vi "AOD Control (FPGA).vi"() -> ()   [LabVIEW 2014]
uses:
  FPGAState.ctl
  AODCalibration.ctl
  CoordinateSettings.ctl
  <vilib>/Platform/TimedLoop/XDataNode/timing_clust.ctl
  <vilib>/Platform/TimedLoop/XDataNode/nitl_modes.ctl
  <vilib>/Platform/TimedLoop/XDataNode/wakeup.ctl
  <vilib>/rvi/Emulation/niFpgaSctlEmulationGetInTimedLoop.vi
  <vilib>/rvi/Emulation/niFpgaEmulationReportErrorSimple.vi
  <vilib>/rvi/Emulation/niFpgaGetClockAttributes.vi
  <vilib>/rvi/Emulation/niFpgaCriticalErrorInLSC.vi
  <vilib>/rvi/eio/common/nirviEmuTemplateMethod_errors.vi
  <vilib>/rvi/Emulation/niFpgaProcessEmulError.vi
  <vilib>/rvi/interface/RandomDataEmulation/niFpgaRandomDataHandleErrors.vi
  <vilib>/Platform/TimedLoop/XDataNode/XDataNode.xnode
  <vilib>/eio/EIONode/EIONode.xnode
  <vilib>/rvi/DataTransferAndStorage/Container/XNode/niFpgaContainer.xnode
  <vilib>/rvi/interface/RandomDataEmulation/nirviRandomDataFpgaReadWriteTemplate.vi
  <vilib>/Platform/TimedLoop/XDataNode/XDNodeRunTimeDep.lvlib
  <vilib>/rvi/occurrence/nirviOccurrence.lvlib
  <vilib>/rvi/Analysis/measure/butterworth/XNode/niFpgaButterworthFilter.xnode
panel:
  out "Status.MotionCorrectionChFull":bool
  out "Status.RelativeRate":u64
  out "Status.Update IO Missing":bool
  out "Status.Last Point":bool
  out "Status.All Samples":bool
  out "Status.AcqState":enum16{"Idling", "Acquiring"}(ring)
  out "Status.TemporalChFull":bool
  out "Status.MotionChFull":bool
  out "Status.ImChFull":bool
  out "Status.BufferedPoints":i32
  out "Status.Sequencer":T1
  out "Status.Initialized":bool
  out "Status.RepNum":u32
  out "Status.Mode":enum16{"Points", "Volume", "Idle"}(ring)
  out "Status.ScanDone":bool
  out "Status.Armed":bool
  out "Status.ScanUpdateIO":bool
  out "Status.Writing":bool
  out "Status.PointTime":u32
  out "Status.PointNum":u32
  out "Status.Sequencing error":bool
  in  "OutOffset.Z":i32
  in  "OutOffset.Y":i32
  in  "OutOffset.X":i32
  in  "InOffset.Z":i32
  in  "InOffset.Y":i32
  in  "InOffset.X":i32
  in  "Setup.DataSource":i16
  in  "Setup.BitShift":i16
  in  "Setup.Downsample":u32=1000
  in  "Setup.Timeout":i32=40000000
  out "Filtered Data":i32[](array[numeric])
  in  "scaled coefficients":i32[](array[numeric])=[-807278098, 1858776710, 5560803, -954717605, 2004472733, 5996674]
  out "Debug.FilterTime":u32
  out "Debug.WriteTime":u32
  out "Debug.Sequencing offset":u32
  in  "Debug.Data":i16
  out "Debug.Settings":T2 {"YLP_RR" format="%x"; "YLP_FR" format="%x"; "YHP_RR" format="%x"; "YHP_FR" format="%x"; "XLP_RR" format="%x"; "XLP_FR" format="%x"; "XHPstart" format="%x"; "XHPend" format="%x"; "XLPstart" format="%x"; "XLPend" format="%x"; "YHPstart" format="%x"; "YHPend" format="%x"; "YLPstart" format="%x"; "YLPend" format="%x"; "XHP_RR" format="%x"; "XHP_FR" format="%x"}
  out "Debug.PMT_Unpacked_backlog":u32
  out "Debug.PMT_Data_backlog":u32
  in  "Debug.FinishedSettingSize":i16=3
  in  "Debug.FinishedSetting":cluster{"Address":u8, "Value":u32}[](array[cluster])=[{"Address"=0, "Value"=246}, {"Address"=4, "Value"=0}, {"Address"=5, "Value"=0}, {"Address"=0, "Value"=0}, {"Address"=0, "Value"=0}] {"Address" format="%x"; "Value" format="%x"}
  in  "Debug.Coordinate":T3
  in  "Debug.SetCoordinate":bool
  out "Debug.AcqDivCount":u32
  out "Debug.PMT_Samples":u32
  out "Debug.MainLoopCount":i32
  in  "Debug.UpdateIO":bool
  out "Debug.PMT Array":i32[](array[numeric])
  in  "Debug.P":bool
  in  "Debug.Point":cluster{"X":i32, "Y":i32, "Z":i32}
  in  "Debug.Write Point":bool
  out "Error.Sequencer":bool
  out "Error.UpdateIOTimeout":bool
  out "Error.Serial error":bool
  out "Error.OutOfRange":bool
  out "Error.Bad Coordinate":bool
  out "Status.WaitingDownsamplerEnd":bool
  in  "Comm.P delay":u32=10
  in  "Comm.P high":u32=10
  in  "Comm.Pause":u32
  in  "Comm.WriteSize":i32
  in  "Comm.Write":cluster{"Address":u8, "Value":u32}[](array[cluster])=[{"Address"=0, "Value"=0}, {"Address"=0, "Value"=0}, {"Address"=0, "Value"=0}, {"Address"=0, "Value"=0}, {"Address"=0, "Value"=0}, {"Address"=0, "Value"=0}, {"Address"=0, "Value"=0}, {"Address"=0, "Value"=0}, {"Address"=0, "Value"=0}, {"Address"=0, "Value"=0}, {"Address"=0, "Value"=0}, {"Address"=0, "Value"=0}, {"Address"=0, "Value"=0}, {"Address"=0, "Value"=0}, {"Address"=0, "Value"=0}, {"Address"=0, "Value"=0}, {"Address"=0, "Value"=0}, {"Address"=0, "Value"=0}, {"Address"=0, "Value"=0}, {"Address"=0, "Value"=0}]
  out "Comm.WritenCount":i32
  in  "Comm.Write Register":bool
  in  "Comm.SclkDivider":u32=10
  in  "Comm.CommLines":enum16{"1", "2", "4"}(ring)
  in  "Comm.UpdateIO time":u32=2
  out "Scan.SampleToLoad":u32
  out "Scan.UpdateIO counter":u32
  out "Scan.Downsample Counter":u32
  in  "Scan.NumMotionPoints":u32
  in  "Scan.Motion Increment":u32
  in  "Scan.TotalSamples":u32
  in  "Scan.VolumeSettings":T4={"XStart"=0, "XEnd"=0, "XNum"=1, "YStart"=0, "YEnd"=0, "YNum"=1, "ZStart"=0, "ZEnd"=0, "ZNum"=1} {"ZNum" min=1 max=10000; "YNum" min=1 max=10000; "XNum" min=1 max=10000}
  in  "Scan.NumReps":i32=1
  in  "Scan.NumPoints":u32
  out "Scan.Acquire Samples":u32
  out "Clock100 PLL Unlocked":bool
  out "IO Module\\Initialization Done":bool
  in  "IO Module\\Force Initialization":bool
  in  "IO Module\\Sample Clock Select":u8
  out "IO Module\\Pll Unlocked":bool
  out "Analog Data":i16[](array[numeric])
  in  "AOD.Calibration":T5={"XHP ChirpGain"=1.0, "YHP ChirpGain"=1.0, "XLP ChirpGain"=1.0, "YLP ChirpGain"=1.0}
  in  "AOD.ThrowawaySamples":u16=40
  in  "AOD.LP Center Frequency":u32=858993459 format="%x"
  in  "AOD.HP Center Frequency":u32=805306367 format="%x"
  in  "AOD.Range":u32=214748364 format="%x"
  in  "AOD.BlankSamples":u16=500
  in  "AOD.UpdatesPerPoint":u32=2000
  in  "Control.Points":bool
  in  "Control.Reset":bool
  in  "Control.Abort":bool
  in  "Control.Volume":bool
  in  "Control.Stop":bool
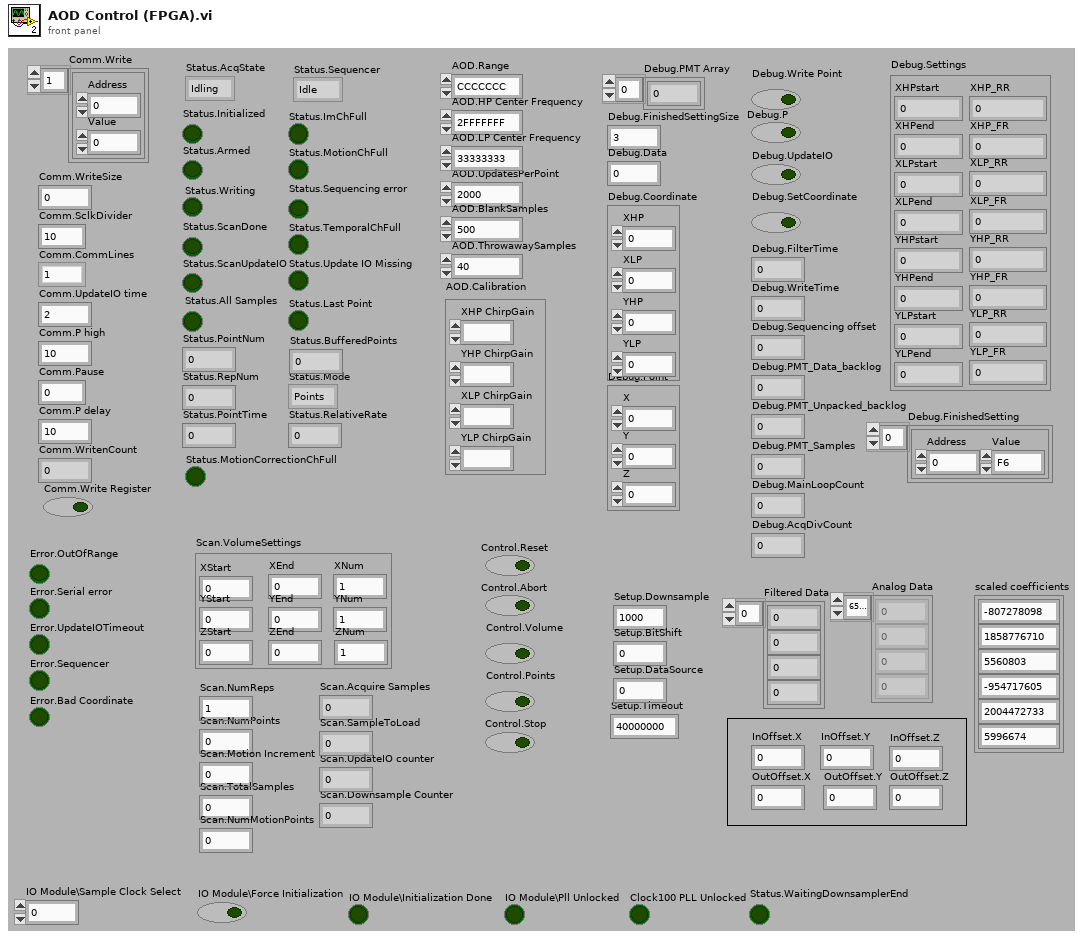
[diagram p1: front panel]
types:
  T1 = typedef "FPGAState.ctl" = enum16{"Idle", "Arm Scan", "Scan", "End Scan"}
  T2 = typedef "CoordinateSettings.ctl" = cluster{"XHPstart":u32, "XHPend":u32, "XLPstart":u32, "XLPend":u32, "YHPstart":u32, "YHPend":u32, "YLPstart":u32, "YLPend":u32, "XHP_RR":u32, "XHP_FR":u32, "XLP_FR":u32, "XLP_RR":u32, "YHP_FR":u32, "YHP_RR":u32, "YLP_FR":u32, "YLP_RR":u32}
  T3 = cluster{"XHP":i32, "XLP":i32, "YHP":i32, "YLP":i32}
  T4 = cluster{"XStart":i32, "XEnd":i32, "XNum":i32, "YStart":i32, "YEnd":i32, "YNum":i32, "ZStart":i32, "ZEnd":i32, "ZNum":i32}
  T5 = typedef "AODCalibration.ctl" = cluster{"XHP ChirpGain":fxp<+/-,16,2>, "YHP ChirpGain":fxp<+/-,16,2>, "XLP ChirpGain":fxp<+/-,16,2>, "YLP ChirpGain":fxp<+/-,16,2>}
  T6 = typedef "XDNodeRunTimeDep.lvlib/timing_clust.ctl" = cluster{"Expected End [f-1]":u64, "Actual End [f-1]":u64, "Finished Late? [f-1]":bool, "Expected End [i-1]":u64, "Actual End [i-1]":u64, "Finished Late? [i-1]":bool, "Expected Start [i]":u64, "Actual Start [i]":u64, "Expected Start [f]":u64, "Actual Start [f]":u64, "Source Name":string, "Structure Name":string, "Period":i64, "Deadline":i64, "Offset":i64, "Start":i64, "Priority":i32, "Timeout":i32, "Mode":T7, "Wakeup Reason":T8, "Error":errorcluster, "Source Type":string, "Secondary Source Type":string, "Global End Time":u64, "Global Start Time":u64, "Frame Duration":u64, "Iteration Duration":u64, "Assigned CPU":i32, "I/O Scan Engine Mode":u32}
  T7 = typedef "XDNodeRunTimeDep.lvlib/nitl_modes.ctl" = enum32{"No Change", "Process missed periods, maintain original phase", "Discard missed periods, maintain original phase", "Process missed periods, ignore original phase", "Discard missed periods, ignore original phase"}
  T8 = typedef "XDNodeRunTimeDep.lvlib/wakeup.ctl" = enum32{"Normal", "Aborted", "Asynchronous wakeup", "Timing source error", "Timed loop error", "Timeout"}
  T9 = cluster{"Scan mode":enum16{"Points", "Volume", "Idle"}, "NumPoints":u32, "NumReps":u32, "Motion Increment":u32, "NumMotionPoints":u32, "VolumeSettings":cluster{"XStart":i32, "XEnd":i32, "XNum":i32, "YStart":i32, "YEnd":i32, "YNum":i32, "ZStart":i32, "ZEnd":i32, "ZNum":i32}}
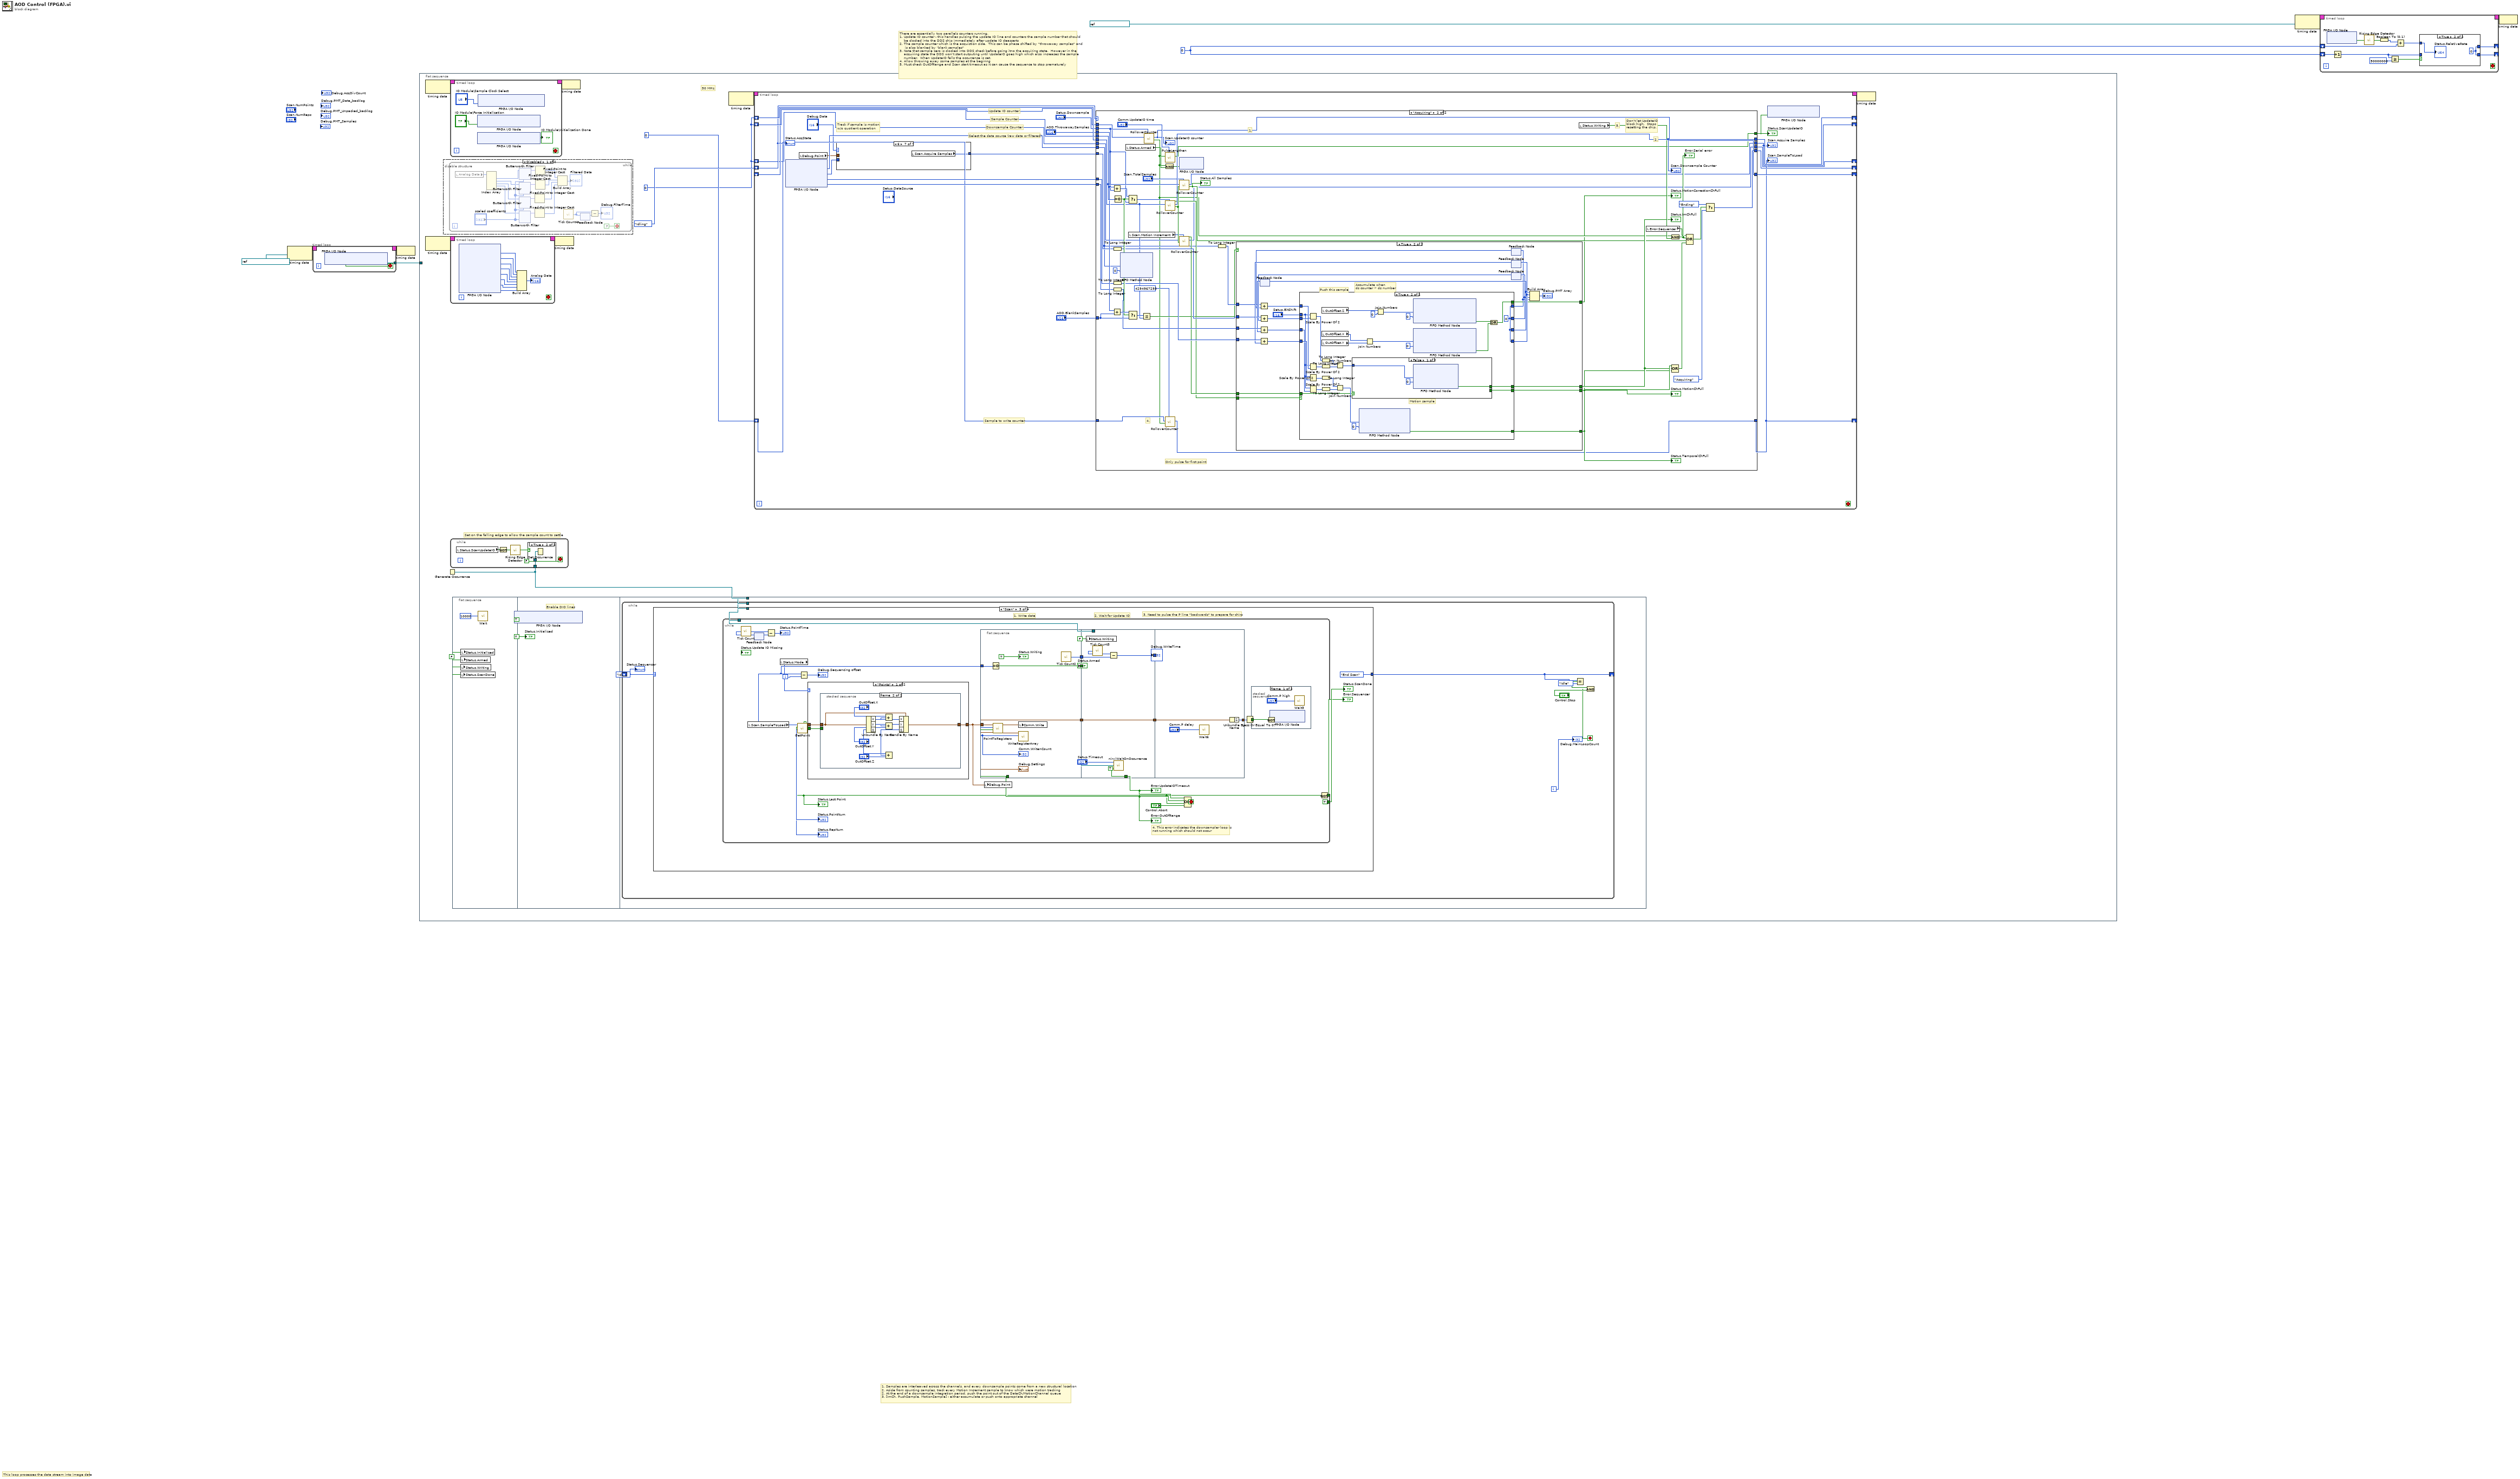
[diagram p0: block diagram]
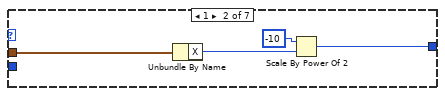
[diagram p6: hidden frame]
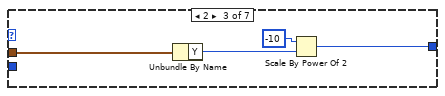
[diagram p7: hidden frame]
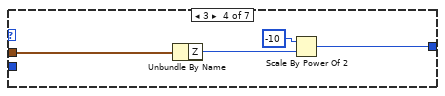
[diagram p8: hidden frame]
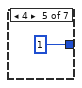
[diagram p9: hidden frame]
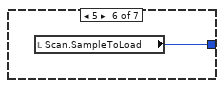
[diagram p10: hidden frame]
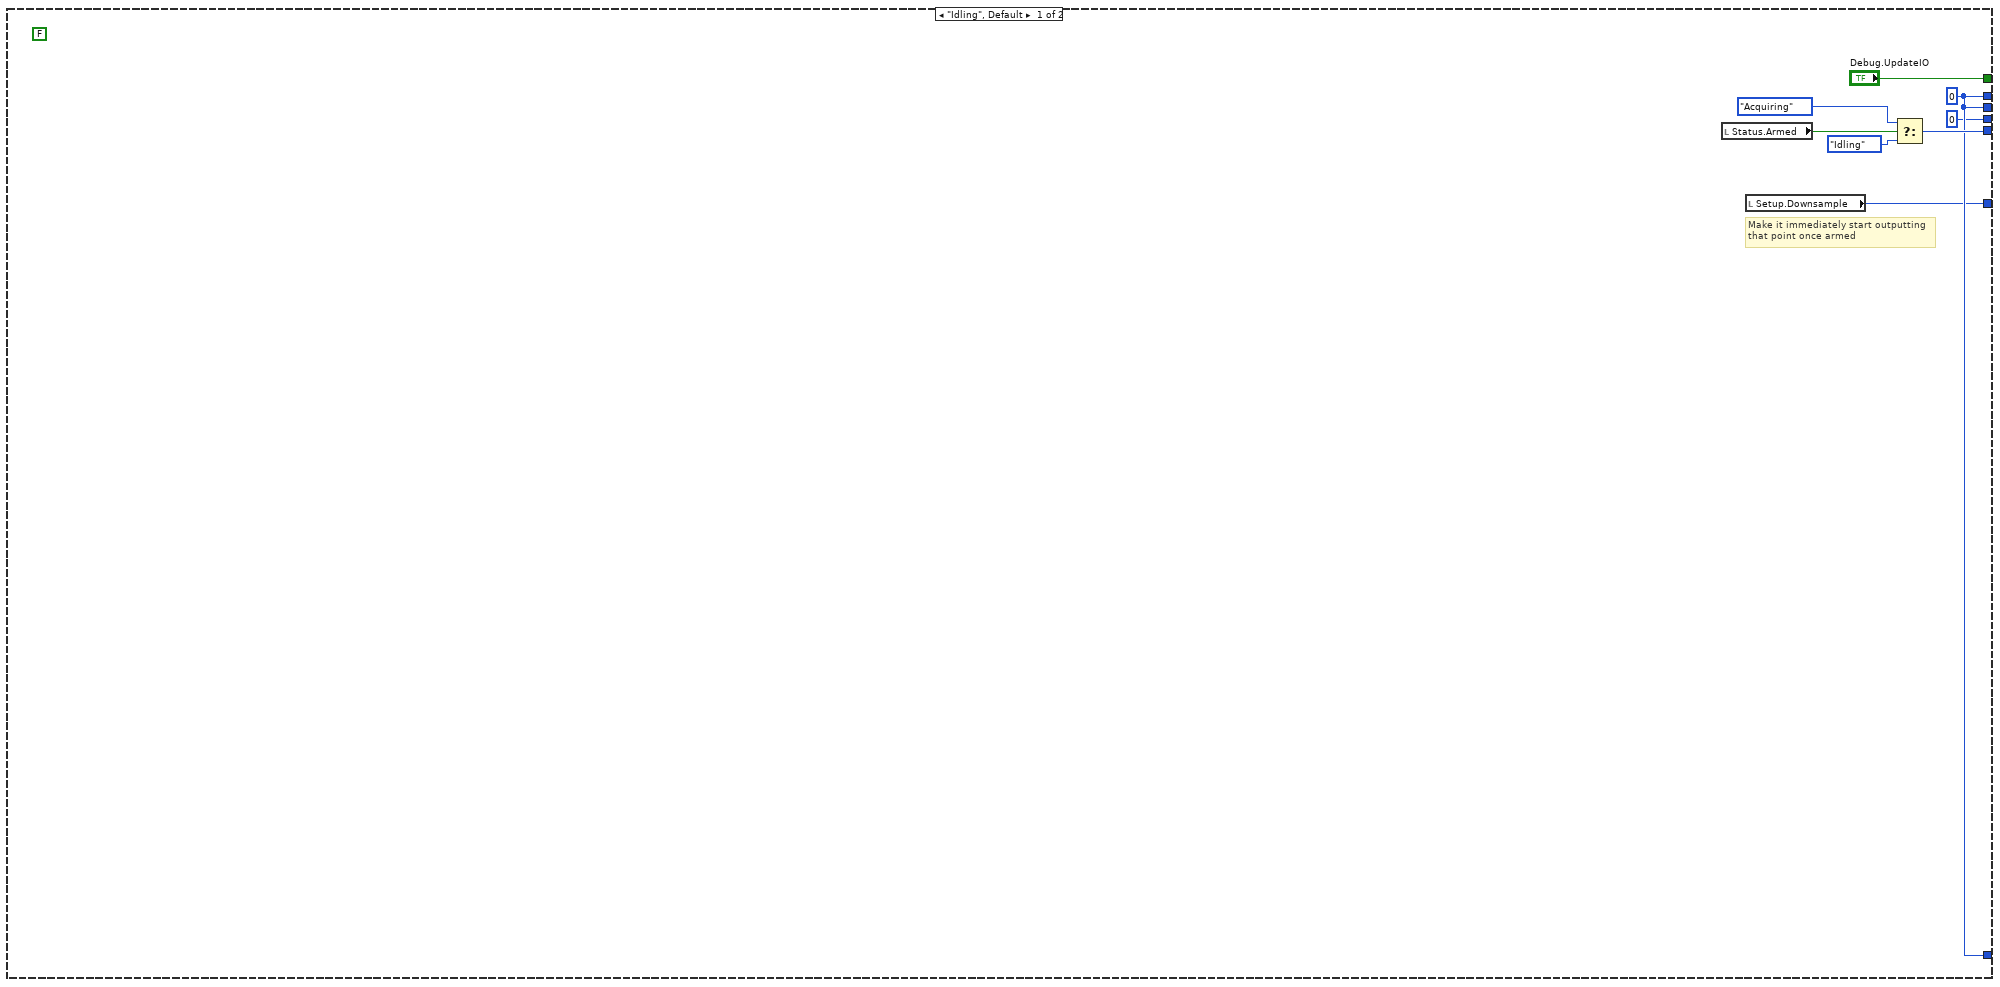
[diagram p11: hidden frame]
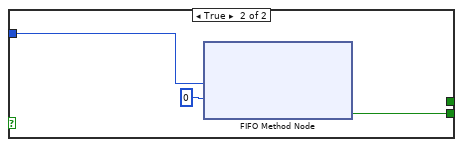
[diagram p14: hidden frame]
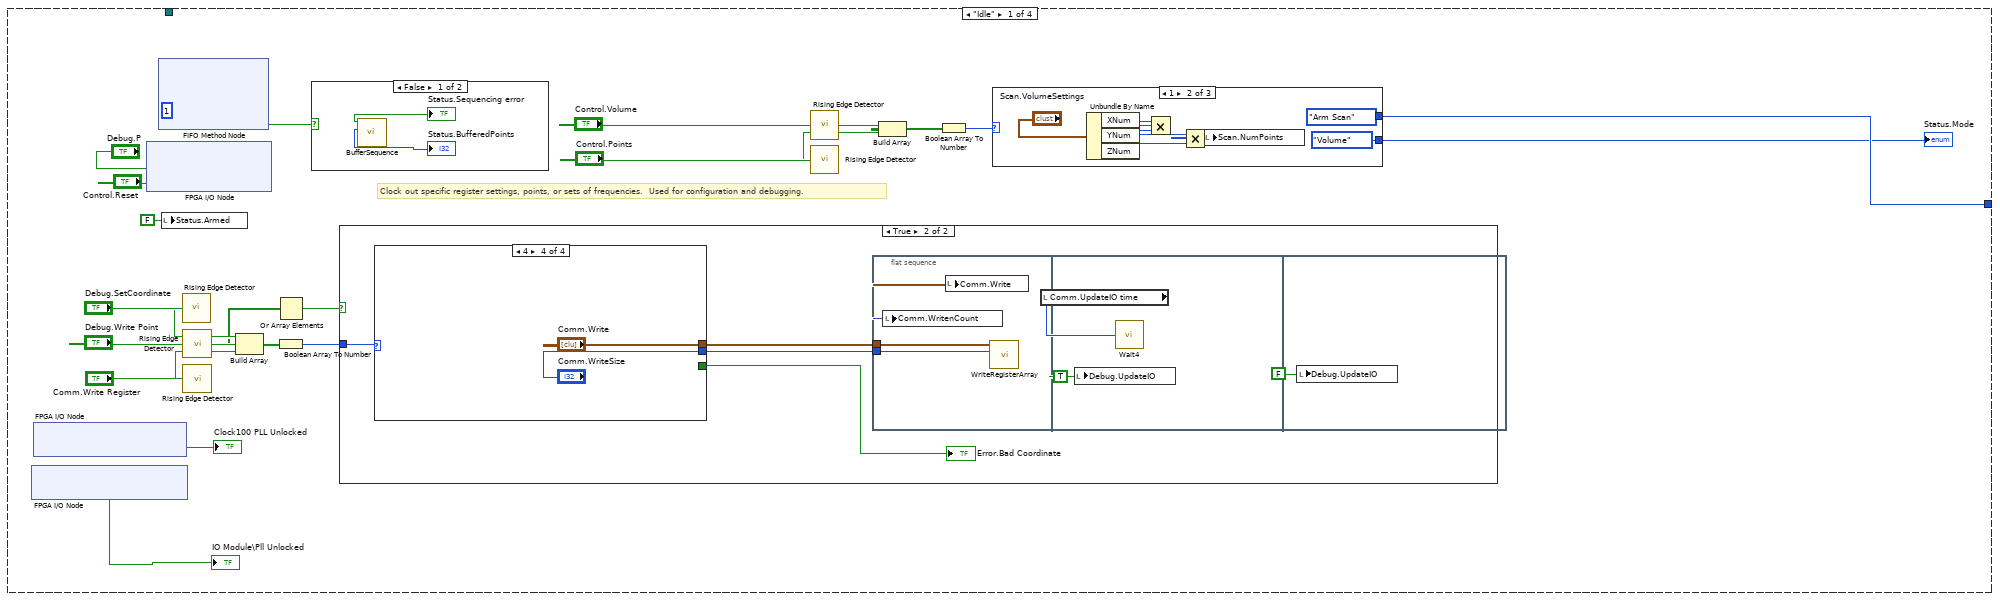
[diagram p15: hidden frame]
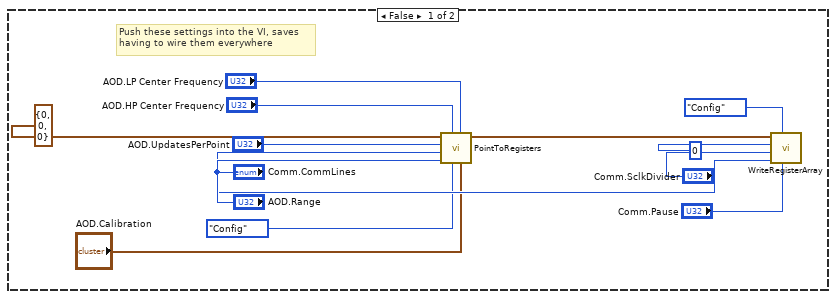
[diagram p17: hidden frame]
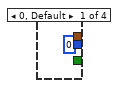
[diagram p18: hidden frame]
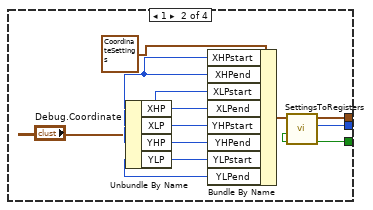
[diagram p19: hidden frame]
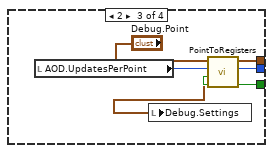
[diagram p20: hidden frame]
diagram:
  w1 = u64 0
  # "There are essentially two parallels counters running.\n1. Update IO counter - this handles pulsing the update IO line and counters the sample number that should\n    be clocked into the DDS chip immediately after update IO deasserts\n2. The sample counter which is the acquistion side.  This can be phase shifted by \"throwaway samples\" and\n     is also blanked by 'blank samples\"\n3. Note that sample zero is clocked into DDS check before going itno the acquiring state.  However in the \n    acquiring state the DDS won't start outputing until UpdateIO goes high which also increases the sample\n    number.  When UpdateIO falls the occurrence is set.\n4. Allow throwing away some samples at the beginng\n5. Must check OutOfRange and Scan start timeout as it can cause the sequence to stop prematurely"
  # "1. Samples are interleaved across the channels, and every downsample points come from a new structural location\n2. Aside from counting samples, track every Motion Increment sample to know which were motion tracking\n2. At the end of a downsample integration period, push the point out of the DataCh/MotionChannel queue\n3. [ImCh, PushSample, MotionSample] - either accumulate or push onto appropriate channel"
  # "This loop processes the data stream into image data"
  n1 = node-c288(refnum<k21> "40 MHz Onboard Clock" ("Source Name")) -> (w8:T6)
  n2 = timed-loop {
    timing: w8 -> [_]
    timing-out: [_] -> w7
    tunnel: [w9] -> w5
    stop <- w10 stop-if-true
    n3 = xnode "FPGA I/O Node"() -> ("IO Module\\Initialization Done"=w10:bool, "FPGA I/O Out"=w9:refnum<k21>)  [unwired: 1 in]
  }
  n4 = node-c288(w7) -> ()
  n5 = flat-sequence {
    tunnel: w5 -> [_]
    frame #0 {
      w13 = u32 0
      # "Set on the falling edge to allow the sample count to settle"
      # "50 MHz"
      n6 = node-c288() -> (w18:T6)  [unwired: 1 in]
      n7 = node-c288() -> (w20:T6)  [unwired: 1 in]
      n8 = disable-structure shown="Disabled" {
        frame Disabled {
          n9 = while {
            stop <- FALSE stop-if-true
            n10 = local read "Analog Data"() -> (w27:i16[])
            n11 = Index Array(array=w27) -> (element #1=w26:i16, element #2=w25:i16, element #3=w24:i16, element #4=w23:i16)  [unwired: 5 in, 1 out]
            n12 = xnode "Butterworth Filter"("input data"=w25, "scaled coefficients"="scaled coefficients") -> ("output data"=w35:fxp<+/-,20,20>)  [unwired: 1 in]
            n13 = xnode "Butterworth Filter"("input data"=w24, "scaled coefficients"="scaled coefficients") -> ("output data"=w34:fxp<+/-,20,20>)  [unwired: 1 in]
            n14 = xnode "Butterworth Filter"("input data"=w23, "scaled coefficients"="scaled coefficients") -> ("output data"=w33:fxp<+/-,20,20>)  [unwired: 1 in]
            n15 = xnode "Butterworth Filter"("input data"=w26, "scaled coefficients"="scaled coefficients") -> ("output data"=w36:fxp<+/-,20,20>)  [unwired: 1 in]
            n16 = Fixed-Point to Integer Cast(1:w34) -> (0:w30:i32)
            n17 = Fixed-Point to Integer Cast(1:w33) -> (0:w29:i32)
            n18 = Fixed-Point to Integer Cast(1:w36) -> (0:w32:i32)
            n19 = Fixed-Point to Integer Cast(1:w35) -> (0:w31:i32)
            n20 = Build Array(w32, w31, w30, w29) -> (→"Filtered Data":i32[])
            n21 = call "Tick Count4"() -> ("Tick Count(Ticks)"=w41:u32)
            n22 = feedback #1() -> (w40:u32)  [unwired: 1 in]
            n23 = feedback-in #1(w41) -> ()
            n24 = Subtract(x=w41, y=w40) -> (x-y=→"Debug.FilterTime":u32)
          }
        }
        frame Enabled {
        }
      }
      n25 = Generate Occurrence() -> (w14:refnum<k4>)
      n26 = timed-loop {
        timing: w18 -> [_]
        timing-out: [_] -> w17
        stop <- _ stop-if-true
        n27 = xnode "FPGA I/O Node"("IO Module\\Force Initialization"="IO Module\\Force Initialization") -> ()  [unwired: 1 in, 1 out]
        n28 = xnode "FPGA I/O Node"() -> ("IO Module\\Initialization Done"=→"IO Module\\Initialization Done":bool)  [unwired: 1 in, 1 out]
        n29 = xnode "FPGA I/O Node"("IO Module\\Sample Clock Select"="IO Module\\Sample Clock Select") -> ()  [unwired: 1 in, 1 out]
      }
      n30 = timed-loop {
        timing: w20 -> [_]
        timing-out: [_] -> w19
        stop <- _ stop-if-true
        n31 = xnode "FPGA I/O Node"() -> ("IO Module\\AI A0"=w91:i16, "IO Module\\AI A1"=w90:i16, "IO Module\\AI A2"=w89:i16, "IO Module\\AI A3"=w88:i16, "IO Module\\AI A4"=w95:i16, "IO Module\\AI A5"=w94:i16, "IO Module\\AI A6"=w93:i16, "IO Module\\AI A7"=w92:i16)  [unwired: 8 in, 8 out]
        n32 = Build Array(w91, w90, w89, w88, w95, w94, w93, w92) -> (→"Analog Data":i16[])
      }
      n33 = while {
        tunnel: w14 -> [w77]
        stop <- FALSE stop-if-true
        n34 = local read "Status.ScanUpdateIO"() -> (w75:bool)
        n35 = Not(x=w75) -> (.not. x?=w74:bool)
        n36 = call "Rising Edge Detector.vi"("Signal In"=w74) -> ("Edge Detected?"=w78:bool)
        n37 = case shown="True" w78 {
          tunnel: w77 -> [_ w79]
          frame False {
          }
          frame True {
            n38 = Set Occurrence(w79) -> ()
          }
        }
      }
      n39 = flat-sequence {
        tunnel: w14 -> [w273]
        frame #0 {
          w269 = FALSE
          n40 = local write "Status.Writing"(w269) -> ()
          n41 = local write "Status.ScanDone"(w269) -> ()
          n42 = local write "Status.Initialized"(w269) -> ()
          n43 = local write "Status.Armed"(w269) -> ()
          n44 = call "Wait"("Count(uSec)"=u32 10000) -> ()  [unwired: 1 out]
        }
        frame #1 {
          # "Enable DIO lines"
          n45 = xnode "FPGA I/O Node"("IO Module\\Digital Output Enable"=TRUE ("IO Module\\DDCA_DIO0-7_WE")) -> ()  [unwired: 1 in, 1 out]
          "Status.Initialized" <- TRUE ("Status.Initialized")
        }
        frame #2 {
          n46 = while {
            shift-right: [w281] -> _
            shift-left: FPGAState."Idle" ("Ring") -> [w276]
            tunnel: w273 -> [w275]
            i -> [w282]
            stop <- w278 stop-if-true
            n47 = case shown="\"Scan\"" w276 {
              tunnel: [w305 FPGAState."Scan" ("Ring") FPGAState."End Scan" ("Ring") FPGAState."Idle" ("Enum")] -> w281
              tunnel: w275 -> [_ _ w387 _]
              frame "Idle" {
                # "Clock out specific register settings, points, or sets of frequencies.  Used for configuration and debugging."
                n48 = xnode "FPGA I/O Node"() -> ("IO Module\\Pll Unlocked"=→"IO Module\\Pll Unlocked":bool)  [unwired: 1 in, 1 out]
                n49 = xnode "FPGA I/O Node"() -> ("Clock100 PLL Unlocked"=→"Clock100 PLL Unlocked":bool)  [unwired: 1 in, 1 out]
                n50 = xnode "FPGA I/O Node"("IO Module\\P"="Debug.P", "IO Module\\RESET"="Control.Reset") -> ()  [unwired: 2 in, 2 out]
                n51 = xnode ("FIFO Method Node")("Timeout"=1) -> ("Timed Out?"=w291:bool)  [unwired: 1 in, 2 out]
                n52 = local write "Status.Armed"(FALSE ("Status.Armed")) -> ()
                n53 = call "Rising Edge Detector.vi"("Signal In"="Debug.SetCoordinate") -> ("Edge Detected?"=w298:bool)
                n54 = call "Rising Edge Detector.vi"("Signal In"="Debug.Write Point") -> ("Edge Detected?"=w297:bool)
                n55 = call "Rising Edge Detector.vi"("Signal In"="Comm.Write Register") -> ("Edge Detected?"=w292:bool)
                n56 = Build Array(w298, w297, w292) -> (w296:bool[])
                n57 = Or Array Elements(Boolean array=w296) -> (logical OR=w295:bool)
                n58 = Boolean Array To Number(Boolean array=w296) -> (number=w294:u8)
                n59 = case shown="False" w291 {
                  frame False {
                    n60 = call "BufferSequence.vi"() -> ("NumPoints"=→"Status.BufferedPoints":i32, "Sequencing error"=→"Status.Sequencing error":bool)  [unwired: 10 in]
                  }
                  frame True {
                  }
                }
                n61 = case shown="True" w295 {
                  tunnel: w294 -> [_ w325]
                  frame False {
                    # "Push these settings into the VI, saves \nhaving to wire them everywhere"
                    n62 = call "PointToRegisters.vi"("Calibration"="AOD.Calibration", "LP Center Frequency"="AOD.LP Center Frequency", "Mode"=enum16{"Normal", "Config"}."Config", "HP Center Frequency"="AOD.HP Center Frequency", "Range"="AOD.Range", "WriteSize"="Comm.CommLines", "UpdatesPerPoint"="AOD.UpdatesPerPoint", "Point"=cluster{"X":i32, "Y":i32, "Z":i32} {"X"=0, "Y"=0, "Z"=0}) -> ("Register Writes"=w309:cluster{"Address":u8, "Value":u32}[])  [unwired: 3 out]
                    n63 = call "WriteRegisterArray.vi"("Pause"="Comm.Pause", "Mode"=enum16{"Normal", "Config"}."Config", "WriteSize"="Comm.CommLines", "SclkDivider"="Comm.SclkDivider", "NumReg"=i16 0, "Register  Values"=w309) -> ()  [unwired: 6 in]
                  }
                  frame True {
                    n64 = case shown="4" w325 {
                      tunnel: [_ w335 w346 "Comm.Write"] -> w323
                      tunnel: [i16 0 ("WriteLength") w334 w345 "Comm.WriteSize"] -> w324
                      tunnel: [_ w333 w344 _] -> w322
                      frame 0, Default {
                      }
                      frame 1 {
                        n65 = Unbundle By Name("Debug.Coordinate") -> ("XHP"=w341:i32, "XLP"=w340:i32, "YHP"=w339:i32, "YLP"=w338:i32)
                        n66 = Bundle By Name(cluster=T2 {"XHPstart"=0, "XHPend"=0, "XLPstart"=0, "XLPend"=0, "YHPstart"=0, "YHPend"=0, "YLPstart"=0, "YLPend"=0, "XHP_RR"=0, "XHP_FR"=0, "XLP_FR"=0, "XLP_RR"=0, "YHP_FR"=0, "YHP_RR"=0, "YLP_FR"=0, "YLP_RR"=0} ("settings"), "XHPstart"=w341, "XHPend"=w341, "XLPstart"=w340, "XLPend"=w340, "YHPstart"=w339, "YHPend"=w339, "YLPstart"=w338, "YLPend"=w338) -> (w337:T2)
                        n67 = call "SettingsToRegisters.vi"("coordinates"=w337) -> ("OutOfRange"=w333:bool, "size(s)"=w334:i32, "Register Writes"=w335:cluster{"Address":u8, "Value":u32}[])  [unwired: 8 in]
                      }
                      frame 2 {
                        n68 = local read "AOD.UpdatesPerPoint"() -> (w347:u32)
                        n69 = call "PointToRegisters.vi"("UpdatesPerPoint"=w347, "Point"="Debug.Point") -> ("settings"=w342:T2, "OutOfRange"=w344:bool, "Number Registers"=w345:i16, "Register Writes"=w346:cluster{"Address":u8, "Value":u32}[])  [unwired: 6 in]
                        n70 = local write "Debug.Settings"(w342) -> ()
                      }
                      frame 4 {
                      }
                    }
                    "Error.Bad Coordinate" <- w322
                    n71 = flat-sequence {
                      tunnel: w324 -> [w327]
                      tunnel: w323 -> [w326]
                      frame #0 {
                        n72 = local write "Comm.WritenCount"(w327) -> ()
                        n73 = local write "Comm.Write"(w326) -> ()
                        n74 = call "WriteRegisterArray.vi"("NumReg"=w327, "Register  Values"=w326) -> ()  [unwired: 10 in]
                      }
                      frame #1 {
                        n75 = local read "Comm.UpdateIO time"() -> (w329:u32)
                        n76 = local write "Debug.UpdateIO"(TRUE ("UpdateIO")) -> ()
                        n77 = call "Wait4"("Count(Ticks)"=w329) -> ()  [unwired: 1 out]
                      }
                      frame #2 {
                        n78 = local write "Debug.UpdateIO"(FALSE ("UpdateIO")) -> ()
                      }
                    }
                  }
                }
                n79 = call "Rising Edge Detector.vi"("Signal In"="Control.Volume") -> ("Edge Detected?"=w289:bool)
                n80 = call "Rising Edge Detector.vi"("Signal In"="Control.Points") -> ("Edge Detected?"=w288:bool)
                n81 = Build Array(w289, w288) -> (w287:bool[])
                n82 = Boolean Array To Number(Boolean array=w287) -> (number=w286:u8)
                n83 = case shown="1" w286 {
                  tunnel: [FPGAState."Idle" ("Ring") FPGAState."Arm Scan" ("Ring") FPGAState."Arm Scan" ("Ring")] -> w305
                  tunnel: [enum16{"Points", "Volume", "Idle"}."Idle" ("Mode") enum16{"Points", "Volume", "Idle"}."Volume" ("Mode") enum16{"Points", "Volume", "Idle"}."Points" ("Mode")] -> w302
                  frame 0, Default {
                    (unwired) 0 ("BufferedPoints")
                  }
                  frame 1 {
                    n84 = Unbundle By Name("Scan.VolumeSettings") -> ("XNum"=w357:i32, "YNum"=w356:i32, "ZNum"=w354:i32)
                    n85 = Multiply(x=w357, y=w356) -> (x*y=w355:i32)
                    n86 = Multiply(x=w355, y=w354) -> (x*y=w352:i32)
                    n87 = local write "Scan.NumPoints"(w352) -> ()
                  }
                  frame 2 {
                  }
                }
                "Status.Mode" <- w302
              }
              frame "Arm Scan" {
                w383 = T9 {"Scan mode"=enum."Points", "NumPoints"=0, "NumReps"=0, "Motion Increment"=0, "NumMotionPoints"=0, "VolumeSettings"={"XStart"=0, "XEnd"=0, "XNum"=1, "YStart"=0, "YEnd"=0, "YNum"=1, "ZStart"=0, "ZEnd"=0, "ZNum"=1}}  # Settings
                w362 = FALSE ("ScanDone")
                # "This logic is a little confusing, and definitely got me for a bit.  Because every M (motionIncrement) point is motion and not a scan point\nscan samples = (M-1)/M * total samples\ntotal samples = M/(M-1) * scan samples\ntotal samples = scan samples + scan samples / (M-1)\nHowever, on top of this, because the terminate logic only looks at if the last point was the last in the point sequence, if the number of\npoints modulo (M-1) is zero, there will be one less motion point than expected."
                n88 = local read "Scan.NumPoints"() -> (w380:u32)
                n89 = local read "Scan.NumReps"() -> (w379:i32)
                n90 = local read "Status.Mode"() -> (w377:enum16{"Points", "Volume", "Idle"})
                n91 = Multiply(x=w380, y=w379) -> (x*y=w373:u32)
                n92 = Decrement(x="Scan.Motion Increment") -> (x-1=w371:u32)
                n93 = Quotient & Remainder(x=w373, y=w371) -> (x-y*floor(x/y)=w370:u32, floor(x/y)=w364:u32)
                n94 = Equal To 0?(x=w364) -> (x = 0?=w369:bool)
                n95 = Not Equal?(x=w377, y=enum16{"Points", "Volume", "Idle"}."Points") -> (x != y?=w368:bool)
                n96 = Equal To 0?(x=w370) -> (x = 0?=w366:bool)
                n97 = Decrement(x=w364) -> (x-1=w365:u32)
                n98 = local read "Scan.VolumeSettings"() -> (w381:T4)
                n99 = Select(t=w365, s=w366, f=w364) -> (s? t:f=w363:u32)
                n100 = Or(x=w368, y=w369) -> (x .or. y?=w367:bool)
                n101 = Add(x=w373, y=w363) -> (x+y=w375:u32)
                n102 = Select(t=w373, s=w367, f=w375) -> (s? t:f=w374:u32)
                n103 = local write "Scan.TotalSamples"(w374) -> ()
                n104 = Bundle By Name(cluster=w383, "Scan mode"=w377, "NumPoints"=w380, "NumReps"=w379, "Motion Increment"="Scan.Motion Increment", "NumMotionPoints"="Scan.NumMotionPoints", "VolumeSettings"=w381) -> (w382:T9)
                n105 = local write "Status.ScanDone"(w362) -> ()
                n106 = local write "Control.Abort"(w362) -> ()
                n107 = local write "Error.Sequencer"(w362) -> ()
                n108 = local write "Status.Armed"(w362) -> ()
                n109 = call "GetPoint.vi"("Mode"=enum16{"Read", "Configure"}."Configure", "Settings"=w382) -> ()  [unwired: 5 in, 5 out]
              }
              frame "Scan" {
                # "3. Need to pulse the P line \"backwards\" to prepare for chirp"
                # "2. Wait for Update IO"
                # "1. Write data"
                n110 = while {
                  tunnel: [TRUE] -> w388
                  tunnel: w387 -> [w404]
                  tunnel: [w396] -> w386
                  i -> [w400]
                  stop <- w412 stop-if-true
                  # "4. This error indicates the downsampler loop is\nnot running which should not occur"
                  n111 = call "Tick Count"() -> ("Tick Count(Ticks)"=w414:u32)
                  n112 = local read "Scan.SampleToLoad"() -> (w401:u32)
                  n113 = feedback-in #2(w414) -> ()
                  n114 = feedback #2() -> (w413:u32)  [unwired: 1 in]
                  n115 = Subtract(x=w414, y=w413) -> (x-y=→"Status.PointTime":u32)
                  n116 = local read "Status.Mode"() -> (w393:enum16{"Points", "Volume", "Idle"})
                  n117 = call "GetPoint.vi"("Sample Number"=w401) -> ("RepNum"=→"Status.RepNum":u32, "Point Num"=→"Status.PointNum":u32, "Done"=w397:bool, "Point"=w392:cluster{"X":i32, "Y":i32, "Z":i32}, "Frame Start"=w390:bool)  [unwired: 6 in]
                  "Status.Last Point" <- w397
                  n118 = Subtract(x=w401, y=w400) -> (x-y=→"Debug.Sequencing offset":u32)
                  n119 = case shown="\"Points\"" w393 {
                    tunnel: w392 -> [w420 w436]
                    tunnel: [w419 w436] -> w391
                    tunnel: w390 -> [w418 _]
                    frame "Points" {
                      n120 = stacked-sequence {
                        tunnel: w420 -> [_ w429]
                        tunnel: [_ w425] -> w419
                        tunnel: w418 -> [w421 _]
                        frame #0 {
                          n121 = case shown="True" w421 {
                            frame False {
                            }
                            frame True {
                              n122 = local write "OutOffset.X"("InOffset.X") -> ()
                              n123 = local write "OutOffset.Y"("InOffset.Y") -> ()
                              n124 = local write "OutOffset.Z"("InOffset.Z") -> ()
                            }
                          }
                        }
                        frame #1 {
                          n125 = Unbundle By Name(w429) -> ("X"=w435:i32, "Y"=w433:i32, "Z"=w431:i32)
                          n126 = Add(x="OutOffset.X", y=w435) -> (x+y=w428:i32)
                          n127 = Add(x=w433, y="OutOffset.Y") -> (x+y=w427:i32)
                          n128 = Add(x=w431, y="OutOffset.Z") -> (x+y=w426:i32)
                          n129 = Bundle By Name(cluster=w429, "X"=w428, "Y"=w427, "Z"=w426) -> (w425:cluster{"X":i32, "Y":i32, "Z":i32})
                        }
                      }
                    }
                    frame "Volume", Default {
                    }
                  }
                  n130 = flat-sequence {
                    tunnel: w391 -> [w447]
                    tunnel: w401 -> [w446]
                    tunnel: [w445] -> w406
                    tunnel: [w447] -> w405
                    tunnel: [w443] -> w398
                    tunnel: [w442] -> w395
                    tunnel: w406 -> [w456]
                    tunnel: w405 -> [w459]
                    tunnel: w404 -> [w458]
                    tunnel: [w457] -> w403
                    tunnel: [w459] -> w402
                    tunnel: w395 -> [w451]
                    tunnel: [w450] -> w394
                    tunnel: [w462] -> w407
                    tunnel: w402 -> [w462]
                    tunnel: w394 -> [w460]
                    frame #0 {
                      n131 = Equal To 0?(x=w446) -> (x = 0?=w445:bool)
                      n132 = call "PointToRegisters.vi"("Point"=w447) -> ("settings"=→"Debug.Settings":T2, "OutOfRange"=w443:bool, "Number Registers"=w448:i16, "Register Writes"=w441:cluster{"Address":u8, "Value":u32}[])  [unwired: 7 in]
                      "Comm.WritenCount" <- w448
                      n133 = local write "Comm.Write"(w441) -> ()
                      n134 = call "WriteRegisterArray.vi"("NumReg"=w448, "Register  Values"=w441) -> ()  [unwired: 10 in]
                      n135 = call "Tick Count2"() -> ("Tick Count(Ticks)"=w442:u32)
                      "Status.Writing" <- TRUE ("Writing")
                    }
                    frame #1 {
                      n136 = local write "Status.Writing"(FALSE ("Status.Writing")) -> ()
                      n137 = call "Tick Count3"() -> ("Tick Count(Ticks)"=w452:u32)
                      n138 = Subtract(x=w452, y=w451) -> (x-y=w450:u32)
                      n139 = call <vilib>:"nirviWaitOnOccurrence.vi"("ignore previous (T)"=TRUE, "occurrence"=w458, "ticks timeout (-1)"="Setup.Timeout") -> ("timed out"=w457:bool)  [unwired: 2 in]
                      "Status.Armed" <- w456
                    }
                    frame #2 {
                      n140 = call "Wait6"("Count(Ticks)"="Comm.P delay") -> ()  [unwired: 1 out]
                      "Debug.WriteTime" <- w460
                    }
                  }
                  n141 = local write "Debug.Point"(w391) -> ()
                  n142 = Compound Arithmetic op=OR(w403, w398, w397, "Control.Abort") -> (w412:bool)
                  n143 = Unbundle By Name(w407) -> ("Z"=w416:i32)
                  n144 = Less Or Equal To 0?(x=w416) -> (x <= 0?=w415:bool)
                  n145 = stacked-sequence {
                    tunnel: w415 -> [w438 w440]
                    frame #0 {
                      n146 = Not(x=w438) -> (.not. x?=w437:bool)
                      n147 = xnode "FPGA I/O Node"("IO Module\\P"=w437) -> ()  [unwired: 1 in, 1 out]
                      n148 = call "Wait3"("Count(Ticks)"="Comm.P high") -> ()  [unwired: 1 out]
                    }
                    frame #1 {
                      n149 = xnode "FPGA I/O Node"("IO Module\\P"=w440) -> ()  [unwired: 1 in, 1 out]
                    }
                  }
                  n150 = Not(x=w397) -> (.not. x?=w396:bool)
                  "Error.OutOfRange" <- w398
                  "Error.UpdateIOTimeout" <- w403
                }
                "Status.ScanDone" <- w388
                "Error.Sequencer" <- w386
              }
              frame "End Scan" {
                n151 = flat-sequence {
                  tunnel: w463 -> [w470]
                  tunnel: w463 -> [w472]
                  frame #0 {
                    n152 = call "WriteRegisterArray.vi"("NumReg"="Debug.FinishedSettingSize", "Register  Values"="Debug.FinishedSetting") -> ()  [unwired: 10 in]
                  }
                  frame #1 {
                    n153 = while {
                      stop <- w467 continue-if-true
                      n154 = local read "Status.AcqState"() -> (w469:enum16{"Idling", "Acquiring"})
                      n155 = Equal?(x=w469, y=enum16{"Idling", "Acquiring"}."Acquiring") -> (x = y?=w467:bool)
                      "Status.WaitingDownsamplerEnd" <- w467
                    }
                  }
                  frame #2 {
                    n156 = local write "Debug.UpdateIO"(TRUE ("Debug.UpdateIO")) -> ()
                    n157 = call "Wait2"("Count(Ticks)"=w470) -> ()  [unwired: 1 out]
                  }
                  frame #3 {
                    n158 = call "Wait5"("Count(Ticks)"=w472) -> ()  [unwired: 1 out]
                    n159 = local write "Debug.UpdateIO"(FALSE ("Debug.UpdateIO")) -> ()
                  }
                }
                n160 = local read "Comm.UpdateIO time"() -> (w463:u32)
              }
            }
            n161 = Equal?(x=w281, y=FPGAState."Idle" ("Ring")) -> (x = y?=w280:bool)
            n162 = And(x=w280, y="Control.Stop") -> (x .and. y?=w278:bool)
            "Debug.MainLoopCount" <- w282
            "Status.Sequencer" <- w276
          }
        }
      }
      n163 = node-c288(w19) -> ()
      n164 = node-c288(w17) -> ()
      n165 = node-c288() -> (w22:T6)  [unwired: 1 in]
      n166 = timed-loop {
        shift-right: [w104] -> _
        shift-left: w13 -> [w122]
        timing: w22 -> [_]
        timing-out: [_] -> w21
        shift-right: [w121] -> _
        shift-left: w13 -> [w120]
        shift-right: [w116] -> _
        shift-left: enum16{"Idling", "Acquiring"}."Idling" -> [w119]
        shift-right: [w112] -> _
        shift-left: _ -> [w109]
        shift-right: [w108] -> _
        shift-left: i16 0 -> [w110]
        shift-right: [w106] -> _
        shift-left: w13 -> [w107]
        stop <- _ stop-if-true
        # "Select the data source (raw data or filtered)"
        # "Sample to write counter"
        # "Update IO counter"
        # "Track if sample is motion\nw/o quotient operation"
        # "Sample Counter"
        # "Downsample Counter"
        n167 = xnode "FPGA I/O Node"() -> ("IO Module\\AI A0"=w103:i16, "IO Module\\AI A1"=w102:i16, "IO Module\\AI A2"=w118:i16, "IO Module\\AI A3"=w117:i16)  [unwired: 4 in, 4 out]
        n168 = local read "Debug.Point"() -> (w101:cluster{"X":i32, "Y":i32, "Z":i32})
        n169 = case shown="6" "Debug.Data" {
          tunnel: w102 -> [w123 _ _ _ _ _ _]
          tunnel: [w123 w127 w130 w134 1 ("IO Module\\AI A1") w137 w138] -> w111
          tunnel: w101 -> [_ w125 w129 w133 _ _ _]
          frame 0, Default {
          }
          frame 1 {
            n170 = Unbundle By Name(w125) -> ("X"=w124:i32)
            n171 = Scale By Power Of 2(n=i8 -10 ("y"), x=w124) -> (x*2^n=w127:i32)
          }
          frame 2 {
            n172 = Unbundle By Name(w129) -> ("Y"=w128:i32)
            n173 = Scale By Power Of 2(n=i8 -10 ("y"), x=w128) -> (x*2^n=w130:i32)
          }
          frame 3 {
            n174 = Unbundle By Name(w133) -> ("Z"=w132:i32)
            n175 = Scale By Power Of 2(n=i8 -10 ("y"), x=w132) -> (x*2^n=w134:i32)
          }
          frame 4 {
          }
          frame 5 {
            n176 = local read "Scan.SampleToLoad"() -> (w137:u32)
          }
          frame 6 {
            n177 = local read "Scan.Acquire Samples"() -> (w138:u32)
          }
        }
        n178 = case shown="\"Acquiring\"" w119 {
          tunnel: "AOD.BlankSamples" -> [_ w198]
          tunnel: "Setup.Downsample" -> [_ w173]
          tunnel: w122 -> [_ w195]
          tunnel: [w142 w194] -> w121
          tunnel: [w142 w158] -> w104
          tunnel: w120 -> [_ w154]
          tunnel: "AOD.ThrowawaySamples" -> [_ w190]
          tunnel: w103 -> [_ w163]
          tunnel: w111 -> [_ w180]
          tunnel: w118 -> [_ w179]
          tunnel: w117 -> [_ w178]
          tunnel: [w146 w177] -> w116
          tunnel: [w141 w174] -> w112
          tunnel: w109 -> [_ w155]
          tunnel: w110 -> [_ w160]
          tunnel: [w142 w157] -> w108
          tunnel: w107 -> [_ w153]
          tunnel: [u32 0 ("Count") w152] -> w106
          tunnel: ["Debug.UpdateIO" w149] -> w105
          frame "Idling", Default {
            w142 = u32 0 ("Count")
            (unwired) FALSE
            # "Make it immediately start outputting\nthat point once armed"
            n179 = local read "Status.Armed"() -> (w143:bool)
            n180 = local read "Setup.Downsample"() -> (w141:u32)
            n181 = Select(t=enum16{"Idling", "Acquiring"}."Acquiring" ("AcqState"), s=w143, f=enum16{"Idling", "Acquiring"}."Idling" ("AcqState")) -> (s? t:f=w146:enum16{"Idling", "Acquiring"})
          }
          frame "Acquiring" {
            # "5."
            # "4."
            # "Only pulse for first point"
            # "Don't let UpdateIO\nblock high.  Stops \nresetting the chip."
            # "2."
            # "1."
            n182 = Add(x=w190, y=w173) -> (x+y=w196:u32)
            n183 = Add(x=w190, y=w198) -> (x+y=w197:u16)
            n184 = To Long Integer(number=w180) -> (32bit integer=w187:i32)
            n185 = To Long Integer(number=w179) -> (32bit integer=w188:i32)
            n186 = To Long Integer(number=w178) -> (32bit integer=w189:i32)
            n187 = Equal To 0?(x=w195) -> (x = 0?=w191:bool)
            n188 = xnode ("FIFO Method Node")("Element"=w163, "Timeout"=0) -> ()  [unwired: 1 in, 2 out]
            n189 = local read "Status.Armed"() -> (w150:bool)
            n190 = Select(t=w196, s=w191, f=w173) -> (s? t:f=w193:u32)
            n191 = Select(t=w197, s=w191, f=w198) -> (s? t:f=w192:u16)
            n192 = local read "Scan.Motion Increment"() -> (w183:u32)
            n193 = Less Or Equal?(x=w192, y=w154) -> (x <= y?=w181:bool)
            n194 = call "RolloverCounter.vi"("RolloverNum"=w173, "In"=w155) -> ("Rollover"=w151:bool, "Count"=w174:u32)  [unwired: 7 in, 1 out]
            "Scan.UpdateIO counter" <- w174
            n195 = And(x=w151, y=w150) -> (x .and. y?=w164:bool)
            n196 = call "PulseLengthen.vi"("Lengthen"="Comm.UpdateIO time", "Pulse"=w151) -> ("Lengthened"=w149:bool)  [unwired: 9 in]
            n197 = call "RolloverCounter.vi"("RolloverNum"=w193, "In"=w154) -> ("Rollover"=w184:bool, "Count"=w194:u32, "Last"=w175:bool)  [unwired: 7 in]
            "Scan.Downsample Counter" <- w194
            n198 = call "RolloverCounter.vi"("RolloverNum"=u32 4294967295, "Increment"=w151, "In"=w160) -> ("Count"=w157:u32)  [unwired: 6 in, 2 out]
            n199 = xnode "FPGA I/O Node"("TRIG5"=w164) -> ()  [unwired: 1 in, 1 out]
            n200 = call "RolloverCounter.vi"("RolloverNum"="Scan.TotalSamples", "Increment"=w184, "In"=w195) -> ("Rollover"=w166:bool, "Count"=w158:u32)  [unwired: 6 in, 1 out]
            "Status.All Samples" <- w166
            n201 = call "RolloverCounter.vi"("RolloverNum"=w183, "Increment"=w184, "In"=w153) -> ("Count"=w152:u32, "Last"=w182:bool)  [unwired: 6 in, 1 out]
            n202 = To Long Integer(number=w163) -> (32bit integer=w186:i32)
            n203 = case shown="True" w181 {
              tunnel: w186 -> [_ w212]
              tunnel: w187 -> [_ w215]
              tunnel: w188 -> [_ w218]
              tunnel: w189 -> [_ w222]
              tunnel: w175 -> [_ w221]
              tunnel: w182 -> [_ w210]
              tunnel: [_ w203] -> w169
              tunnel: [_ w202] -> w168
              tunnel: [_ w201] -> w167
              tunnel: [_ w199] -> w147
              frame False {
              }
              frame True {
                # "Accumulate when \nds counter > ds number"
                # "Push this sample"
                n204 = feedback #3() -> (w219:i32)  [unwired: 1 in]
                n205 = Add(x=w222, y=w219) -> (x+y=w220:i32)
                n206 = feedback #4() -> (w211:i32)  [unwired: 1 in]
                n207 = Add(x=w212, y=w211) -> (x+y=w213:i32)
                n208 = feedback #5() -> (w216:i32)  [unwired: 1 in]
                n209 = Add(x=w218, y=w216) -> (x+y=w217:i32)
                n210 = feedback #6() -> (w214:i32)  [unwired: 1 in]
                n211 = Add(x=w215, y=w214) -> (x+y=w200:i32)
                n212 = case shown="True" w221 {
                  tunnel: w220 -> [w226 w253]
                  tunnel: [w226 w258] -> w208
                  tunnel: [w225 w258] -> w207
                  tunnel: w217 -> [w225 w254]
                  tunnel: w200 -> [w224 w243]
                  tunnel: [w224 w258] -> w206
                  tunnel: w213 -> [w223 w242]
                  tunnel: [w223 w258] -> w205
                  tunnel: w210 -> [_ w255]
                  tunnel: "Setup.BitShift" -> [_ w241]
                  tunnel: [_ w240] -> w203
                  tunnel: [_ w239] -> w202
                  tunnel: [_ w238] -> w201
                  tunnel: [_ w237] -> w199
                  frame False {
                    # "Blanking.  Could also loop zeros and\naccumulate in here later to clean up \ncode"
                  }
                  frame True {
                    w258 = 0
                    # "Motion sample"
                    n213 = Scale By Power Of 2(n=w241, x=w242) -> (x*2^n=w248:i32)
                    n214 = Scale By Power Of 2(n=w241, x=w243) -> (x*2^n=w247:i32)
                    n215 = Scale By Power Of 2(n=w241, x=w254) -> (x*2^n=w252:i32)
                    n216 = Scale By Power Of 2(n=w241, x=w253) -> (x*2^n=w251:i32)
                    n217 = To Long Integer(number=w248) -> (32bit integer=w246:i32)
                    n218 = To Long Integer(number=w247) -> (32bit integer=w245:i32)
                    n219 = To Long Integer(number=w252) -> (32bit integer=w250:i32)
                    n220 = To Long Integer(number=w251) -> (32bit integer=w249:i32)
                    n221 = local read "OutOffset.Z"() -> (w229:i32)
                    n222 = local read "OutOffset.X"() -> (w228:i32)
                    n223 = local read "OutOffset.Y"() -> (w227:i32)
                    n224 = Join Numbers(hi=w246, lo=w245) -> ((hi.lo)=w244:u64)
                    n225 = Join Numbers(hi=w250, lo=w249) -> ((hi.lo)=w256:u64)
                    n226 = case shown="False" w255 {
                      tunnel: w244 -> [w261 w264]
                      tunnel: [_ w262] -> w240
                      tunnel: [w259 _] -> w239
                      frame False {
                        n227 = xnode ("FIFO Method Node")("Element"=w261, "Timeout"=0) -> ("Timed Out?"=w259:bool)  [unwired: 1 in, 1 out]
                      }
                      frame True {
                        n228 = xnode ("FIFO Method Node")("Element"=w264, "Timeout"=0) -> ("Timed Out?"=w262:bool)  [unwired: 1 in, 1 out]
                      }
                    }
                    n229 = xnode ("FIFO Method Node")("Element"=w256, "Timeout"=0) -> ("Timed Out?"=w238:bool)  [unwired: 1 in, 1 out]
                    n230 = Join Numbers(hi=w228, lo=w227) -> ((hi.lo)=w232:u64)
                    n231 = Join Numbers(hi=w229, lo=0 ("number")) -> ((hi.lo)=w235:u64)
                    n232 = xnode ("FIFO Method Node")("Element"=w235, "Timeout"=0) -> ("Timed Out?"=w230:bool)  [unwired: 1 in, 1 out]
                    n233 = xnode ("FIFO Method Node")("Element"=w232, "Timeout"=0) -> ("Timed Out?"=w231:bool)  [unwired: 1 in, 1 out]
                    n234 = Or(x=w230, y=w231) -> (x .or. y?=w237:bool)
                  }
                }
                n235 = feedback-in #3(w208) -> ()
                n236 = feedback-in #4(w205) -> ()
                n237 = feedback-in #5(w207) -> ()
                n238 = feedback-in #6(w206) -> ()
                n239 = Build Array(w208, w207, w206, w205) -> (→"Debug.PMT Array":i32[])
              }
            }
            "Status.TemporalChFull" <- w167
            "Status.ImChFull" <- w168
            "Status.MotionChFull" <- w169
            "Status.MotionCorrectionChFull" <- w147
            n240 = local read "Status.Writing"() -> (w172:bool)
            n241 = local read "Error.Sequencer"() -> (w148:bool)
            n242 = And(x=w151, y=w172) -> (x .and. y?=w165:bool)
            "Error.Serial error" <- w165
            n243 = Compound Arithmetic op=OR(w169, w168, w167) -> (w156:bool)
            n244 = Compound Arithmetic op=OR(w148, w165, w166, w156) -> (w161:bool)
            n245 = Select(t=enum16{"Idling", "Acquiring", "Ending"}."Ending", s=w161, f=enum16{"Idling", "Acquiring", "Ending"}."Acquiring") -> (s? t:f=w177:enum16{"Idling", "Acquiring", "Ending"})
          }
        }
        "Scan.SampleToLoad" <- w108
        "Status.ScanUpdateIO" <- w105
        "Scan.Acquire Samples" <- w104
        n246 = xnode "FPGA I/O Node"("IO Module\\UPDATE_IO"=w105) -> ()  [unwired: 1 in, 1 out]
        "Status.AcqState" <- w119
      }
      n247 = node-c288(w21) -> ()
    }
  }
  n248 = node-c288(refnum<k21> "IO Module Clock 0" ("Source Name")) -> (w4:T6)
  n249 = timed-loop {
    timing: w4 -> [_]
    timing-out: [_] -> w3
    shift-right: [w478] -> _
    shift-left: w1 -> [w482]
    shift-right: [w477] -> _
    shift-left: w1 -> [w481]
    stop <- _ stop-if-true
    n250 = xnode "FPGA I/O Node"() -> ("PXI_Clk10"=w474:bool)  [unwired: 1 in, 1 out]
    n251 = Increment(x=w481) -> (x+1=w475:u64)
    n252 = call "Rising Edge Detector.vi"("Signal In"=w474) -> ("Edge Detected?"=w484:bool)
    n253 = Boolean To (0,1)(Boolean=w484) -> (0, 1=w483:i16)
    n254 = Greater Or Equal?(x=w475, y=u64 50000000) -> (x >= y?=w479:bool)
    n255 = Add(x=w483, y=w482) -> (x+y=w476:u64)
    n256 = case shown="True" w479 {
      tunnel: [w486 w488] -> w478
      tunnel: [w485 w488] -> w477
      tunnel: w476 -> [w486 w487]
      tunnel: w475 -> [w485 _]
      frame False {
      }
      frame True {
        w488 = i16 0
        "Status.RelativeRate" <- w487
      }
    }
  }
  n257 = node-c288(w3) -> ()
